vi "WPI_CameraSend Images To PC Loop_2Camera.vi"(8 "error in (no error)":errorcluster, 10 "CameraDevRef 2":T1, 11 "CameraDevRef":T1) -> ()   [LabVIEW 2015]
doc: "This VI is used to send images to the dashboard using the second enet port on the 8 slot controller. This is provided for compatibility, but is higher overhead than using the Camera MJPG approach.\n\nThis software is licensed. Open the labview\\readme\\WPI Robotics Library Open Source License.txt file for more information."
uses:
  <vilib>/Rock Robotics/WPI/Camera/WPI_CameraDevRef.ctl
  <vilib>/Rock Robotics/SystemInterfaces/NetworkCommunication/NetComm_UsageReport_ResourceType.ctl
  feed.vi
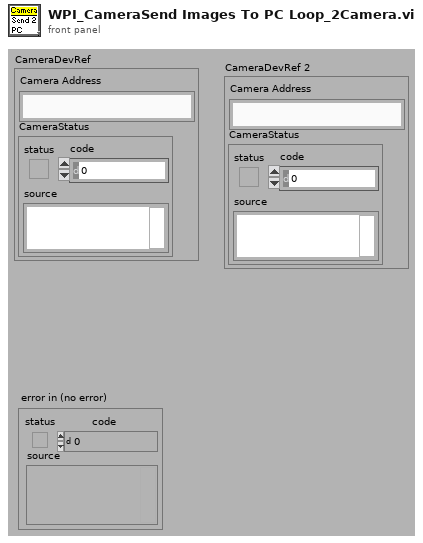
[diagram p1: front panel]
types:
  T1 = typedef "WPI_CameraDevRef.ctl" = cluster{"Camera Address":string, "CameraStatus":errorcluster}
  T2 = cluster{"fps":i32, "compression":i32, "compression 2":i32}
  T3 = typedef "NetComm_UsageReport_ResourceType.ctl" = enum8{"Controller", "Module", "Language", "CANPlugin", "Accelerometer", "ADXL345", "AnalogChannel", "AnalogTrigger", "AnalogTriggerOutput", "CANJaguar", "Compressor", "Counter", "Dashboard", "DigitalInput", "DigitalOutput", "DriverStationCIO", "DriverStationEIO", "DriverStationLCD", "Encoder", "GearTooth", "Gyro", "I2C", "Framework", "Jaguar", "Joystick", "Kinect", "KinectStick", "PIDController", "Preferences", "PWM", "Relay", "RobotDrive", "SerialPort", "Servo", "Solenoid", "SPI", "Task", "Ultrasonic", "Victor", "Button", "Command", "AxisCamera", "PCVideoServer", "SmartDashboard", "Talon", "HiTechnicColorSensor", "HiTechnicAccel", "HiTechnicCompass", "SRF08", "AnalogOutput", "Victor SP", "Talon SRX", "CAN Talon SRX", "ADXL362 Accel", "ADXRS450 Gyro", "Rev SPARK", "Mindsensors SD540", "Digital Filter"}
  T4 = enum16{"Update Mode", "Get Image", "Get Image Data"}
  T5 = typedef "Image Type" = u32
  T6 = typedef "IMAQ Image.ctl" = refnum<image>
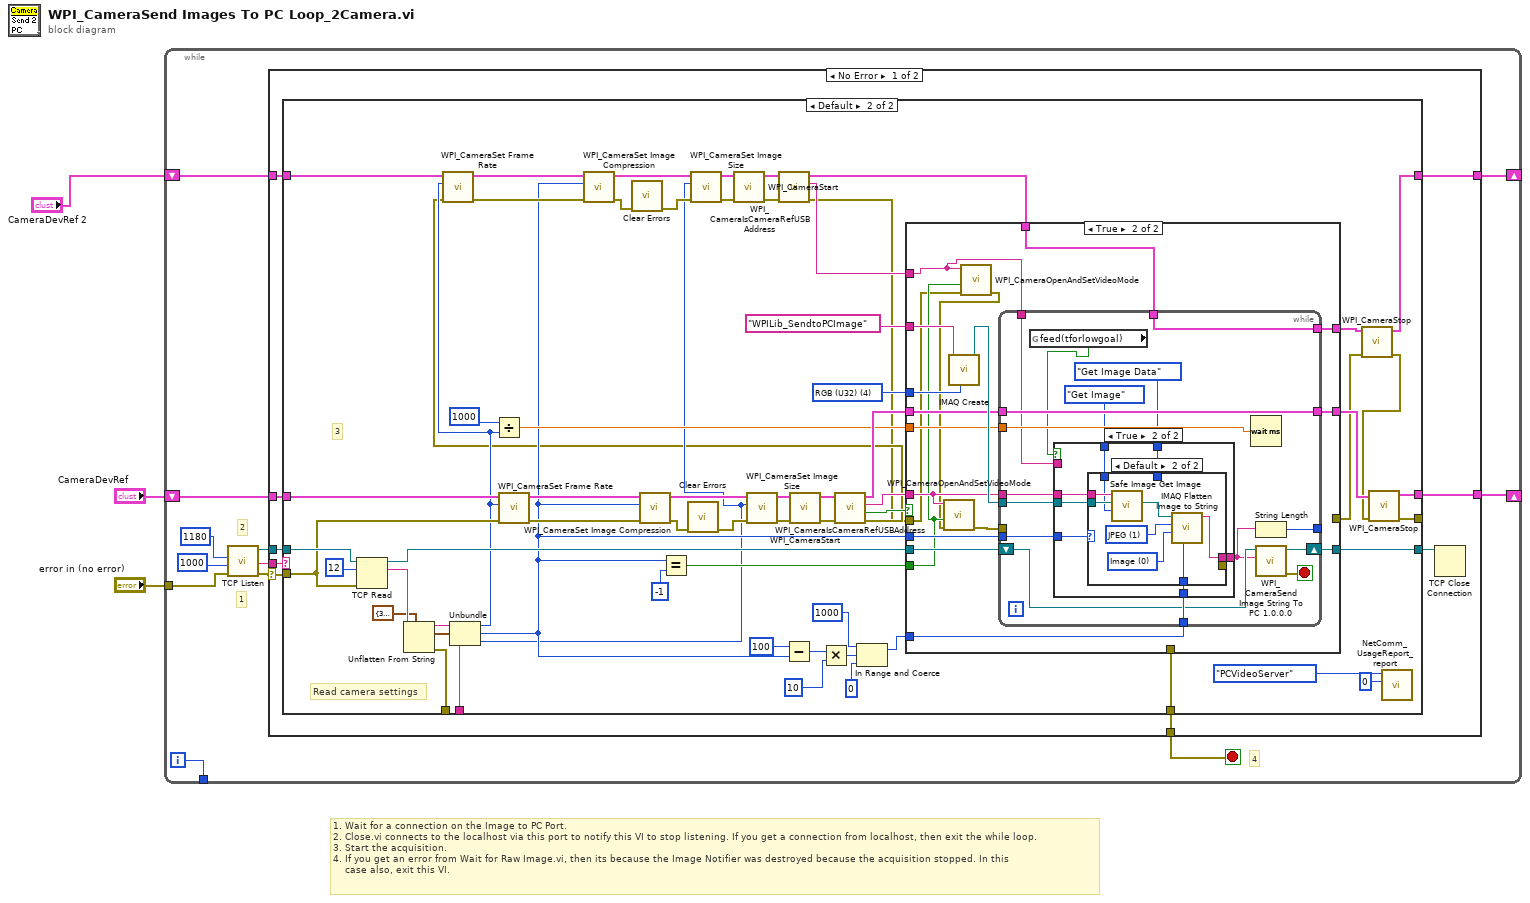
[diagram p0: block diagram]
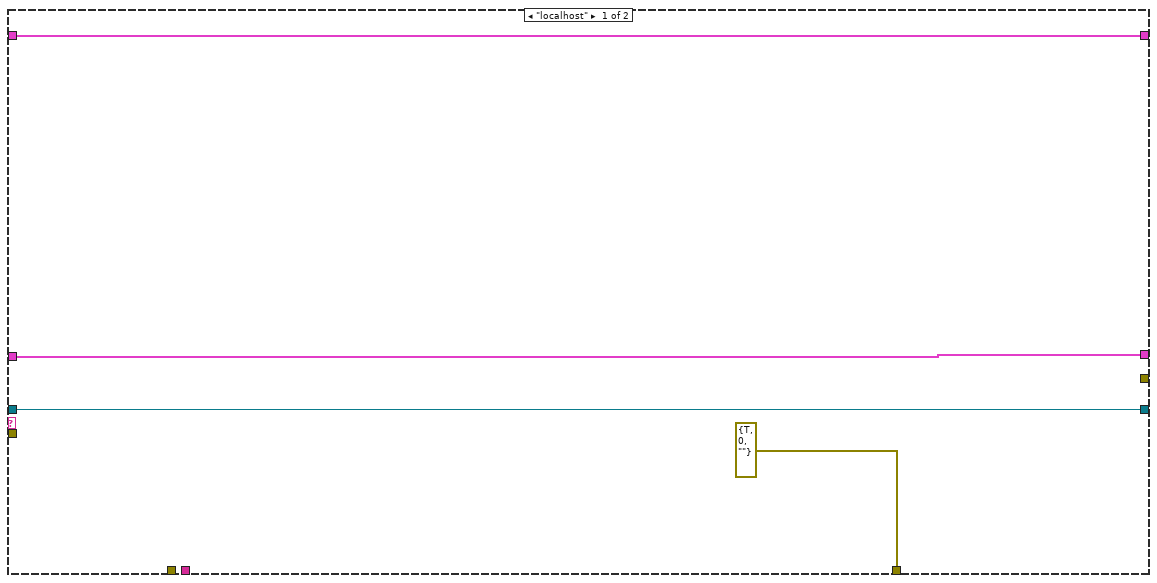
[diagram p2: hidden frame]
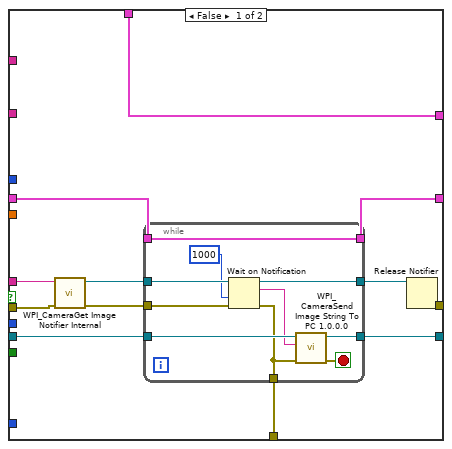
[diagram p3: hidden frame]
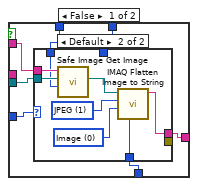
[diagram p4: hidden frame]
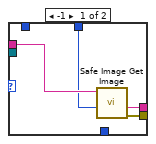
[diagram p5: hidden frame]
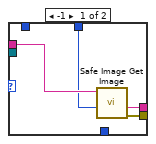
[diagram p6: hidden frame]
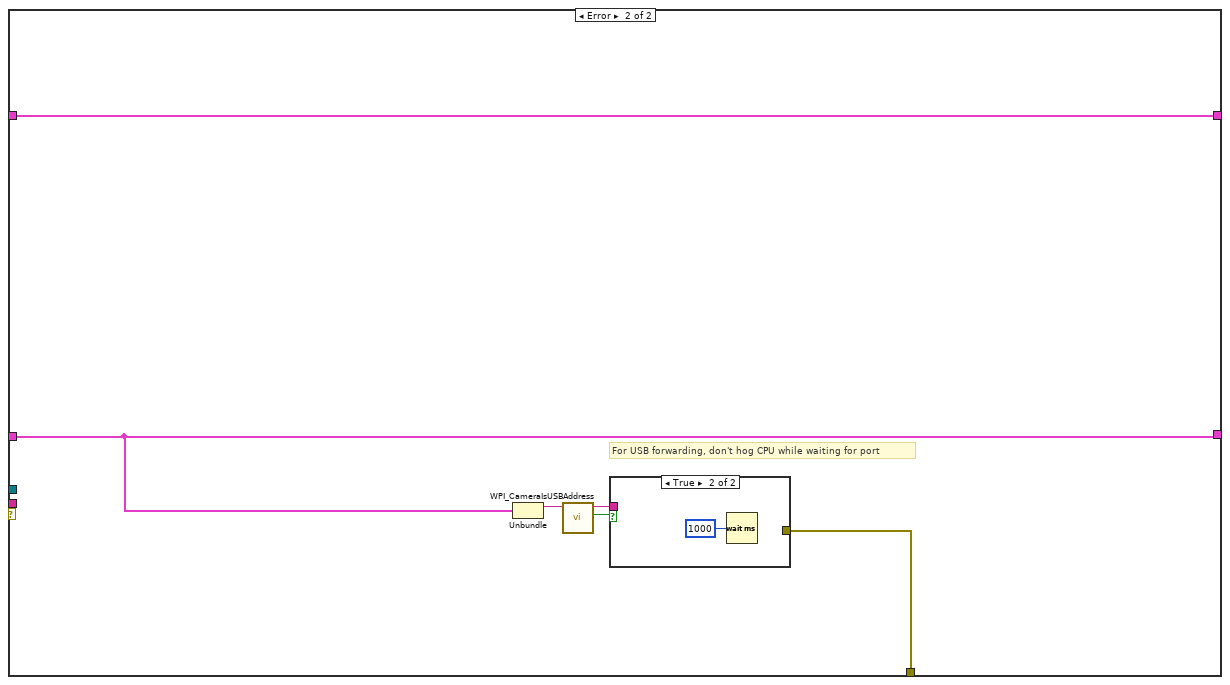
[diagram p7: hidden frame]
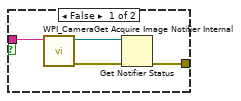
[diagram p8: hidden frame]
diagram:
  # "1. Wait for a connection on the Image to PC Port.\n2. Close.vi connects to the localhost via this port to notify this VI to stop listening. If you get a connection from localhost, then exit the while loop.\n3. Start the acquisition.\n4. If you get an error from Wait for Raw Image.vi, then its because the Image Notifier was destroyed because the acquisition stopped. In this\n    case also, exit this VI."
  n1 = while {
    tunnel: "error in (no error)" -> [w12]
    shift-right: [w15] -> _
    shift-left: "CameraDevRef" -> [w13]
    tunnel: [w6] -> _
    shift-right: [w4] -> _
    shift-left: "CameraDevRef 2" -> [w5]
    i -> [w6]
    stop <- w10 stop-if-true
    # "4"
    # "1"
    # "2"
    n2 = call <vilib>:"TCP Listen.vi"("error in (no error)"=w12, "timeout ms (wait forever: -1)"=u16 1000 ("port"), "port"=u16 1180) -> ("error out"=w8:errorcluster, "remote address"=w14:string, "connection ID"=w11:refnum<k5>)  [unwired: 1 in, 5 out]
    n3 = case shown="No Error" w8 {
      selector: w8 -> [w18 _]
      tunnel: [w24 w190] -> w15
      tunnel: w14 -> [w23 _]
      tunnel: w13 -> [w22 w190]
      tunnel: w11 -> [w21 _]
      tunnel: [w20 w191] -> w10
      tunnel: w5 -> [w17 w186]
      tunnel: [w16 w186] -> w4
      frame No Error {
        n4 = case shown="Default" w23 {
          tunnel: [w28 w89] -> w24
          tunnel: w22 -> [w28 w73]
          tunnel: w18 -> [_ w69]
          tunnel: w21 -> [w26 w77]
          tunnel: [errorcluster {"status"=TRUE, "code"=0, "source"=""} ("error out 2") w91] -> w20
          tunnel: [w26 w90] -> w19
          tunnel: [_ w88] -> _
          tunnel: [_ w51] -> _
          tunnel: [_ w50] -> _
          tunnel: w17 -> [w25 w40]
          tunnel: [w25 w33] -> w16
          frame "localhost" {
          }
          frame Default {
            w83 = T5 4 items=["Grayscale (U8)", "Grayscale (I16)", "Grayscale (SGL)", "Complex (CSG)", "RGB (U32)", "HSL (U32)", "RGB (U64)", "Grayscale (U16)"] ("Image Type")
            # "Read camera settings"
            # "3"
            n5 = TCP Read(connection ID=w77, bytes to read=12, error in (no error)=w69) -> (connection ID out=w76:refnum<k5>, data out=w74:string)  [unwired: 2 in, 1 out]
            n6 = Unflatten From String(type=T2 {"fps"=30, "compression"=32, "compression 2"=32} ("Camera Settings"), binary string=w74) -> (rest of the binary string=w50:string, value=w66:T2, error out=w51:errorcluster)  [unwired: 3 in]
            n7 = Unbundle(w66) -> ("fps"=w38:i32, "compression"=w39:i32, "compression 2"=w37:i32)
            n8 = Divide(x=u16 1000 ("port"), y=w38) -> (x/y=w64:dbl)
            n9 = call <vilib>:"WPI_CameraSet Frame Rate.vi"("error in (no error)"=w69, "Frame Rate (fps)"=w38, "CameraDevRef"=w73) -> ("error out"=w68:errorcluster, "CameraDevRef Out"=w72:T1)  [unwired: 7 in]
            n10 = call <vilib>:"WPI_CameraSet Image Compression.vi"("error in (no error)"=w68, "Compression"=w39, "CameraDevRef"=w72) -> ("error out"=w53:errorcluster, "CameraDevRef Out"=w71:T1)  [unwired: 7 in]
            n11 = Equal?(x=w39, y=-1) -> (x = y?=w54:bool)
            n12 = call <vilib>:"Clear Errors.vi"("error in (no error)"=w53) -> ("error out"=w52:errorcluster)  [unwired: 5 in, 1 out]
            n13 = call <vilib>:"WPI_CameraSet Image Size.vi"("error in (no error)"=w52, "Image Size"=w37, "CameraDevRef"=w71) -> ("error out"=w67:errorcluster, "CameraDevRef Out"=w70:T1)  [unwired: 7 in]
            n14 = Subtract(x=100, y=w39) -> (x-y=w59:i32)
            n15 = call <vilib>:"WPI_CameraStart.vi"("error in (no error)"=w67, "CameraDevRef"=w70) -> ("error out"=w80:errorcluster, "CameraDevRef"=w79:T1)  [unwired: 8 out]
            n16 = Multiply(x=w59, y=10) -> (x*y=w61:i32)
            n17 = call <vilib>:"WPI_CameraIsCameraRefUSBAddress.vi"("error in (no error)"=w80, "CameraDevRef"=w79) -> ("error out"=w32:errorcluster, "USB?"=w81:bool, "Camera Address Out"=w82:string, "CameraDevRef out"=w78:T1)  [unwired: 6 in]
            n18 = call <vilib>:"WPI_CameraSet Frame Rate.vi"("error in (no error)"=w32, "Frame Rate (fps)"=w38, "CameraDevRef"=w40) -> ("error out"=w46:errorcluster, "CameraDevRef Out"=w43:T1)  [unwired: 7 in]
            n19 = call <vilib>:"WPI_CameraSet Image Compression.vi"("error in (no error)"=w46, "Compression"=w39, "CameraDevRef"=w43) -> ("error out"=w48:errorcluster, "CameraDevRef Out"=w44:T1)  [unwired: 7 in]
            n20 = call <vilib>:"Clear Errors.vi"("error in (no error)"=w48) -> ("error out"=w49:errorcluster)  [unwired: 5 in, 1 out]
            n21 = call <vilib>:"WPI_CameraSet Image Size.vi"("error in (no error)"=w49, "Image Size"=w37, "CameraDevRef"=w44) -> ("error out"=w47:errorcluster, "CameraDevRef Out"=w45:T1)  [unwired: 7 in]
            n22 = call <vilib>:"WPI_CameraStart.vi"("error in (no error)"=w47, "CameraDevRef"=w45) -> ("error out"=w41:errorcluster, "CameraDevRef"=w42:T1)  [unwired: 8 out]
            n23 = call <vilib>:"WPI_CameraIsCameraRefUSBAddress.vi"("error in (no error)"=w41, "CameraDevRef"=w42) -> ("error out"=w31:errorcluster, "Camera Address Out"=w36:string, "CameraDevRef out"=w34:T1)  [unwired: 6 in, 1 out]
            n24 = In Range and Coerce(upper limit=1000, x=w61, lower limit=0) -> (coerced(x)=w57:i32)  [unwired: 1 out]
            n25 = case shown="True" w81 {
              tunnel: w76 -> [w103 w131]
              tunnel: [w102 _] -> w91
              tunnel: [w101 w130] -> w90
              tunnel: w31 -> [w100 w114]
              tunnel: w82 -> [w98 w121]
              tunnel: [w97 w125] -> w87
              tunnel: w78 -> [w96 w126]
              tunnel: [w94 _] -> w30
              tunnel: "WPILib_SendtoPCImage" -> [_ w128]
              tunnel: w83 -> [_ w127]
              tunnel: w57 -> [_ w124]
              tunnel: w64 -> [_ w123]
              tunnel: w39 -> [_ w122]
              tunnel: w54 -> [_ w116]
              tunnel: w36 -> [_ w119]
              tunnel: [w92 w118] -> w35
              tunnel: w34 -> [w92 w117]
              frame False {
                n26 = call <vilib>:"WPI_CameraGet Image Notifier Internal.vi"("error in (no error)"=w100, "Camera Address"=w98) -> ("error out"=w99:errorcluster, "Image Notifier"=w95:refnum<notifier>)  [unwired: 8 out]
                n27 = while {
                  tunnel: w99 -> [w109]
                  tunnel: w103 -> [w113]
                  tunnel: [w106] -> w102
                  tunnel: [w111] -> w101
                  tunnel: [w110] -> w97
                  tunnel: w96 -> [w110]
                  tunnel: w95 -> [w108]
                  tunnel: [w104] -> w93
                  stop <- w112 stop-if-true
                  n28 = Wait on Notification(notifier=w108, timeout in ms (-1)=1000 ("Timeout in ms (-1)"), error in (no error)=w109) -> (notifier out=w104:refnum<notifier>, notification=w107:string, error out=w106:errorcluster)  [unwired: 2 out]
                  n29 = call <vilib>:"WPI_CameraSend Image String To PC 1.0.0.0.vi"("error in (no error)"=w106, "String"=w107, "TCP Connection ID"=w113) -> ("error out"=w112:errorcluster, "TCP Connection ID out"=w111:refnum<k5>)  [unwired: 7 out]
                }
                n30 = Release Notifier(notifier=w93) -> (error out=w94:errorcluster)  [unwired: 1 in, 3 out]
              }
              frame True {
                n31 = call "IMAQ Create"("Image Name"=w128, "Image Type"=w127) -> ("New Image"=w129:T6)  [unwired: 3 in, 1 out]
                n32 = call <vilib>:"WPI_CameraOpenAndSetVideoMode.vi"("error in (no error)"=w114, "USB JPEG"=w116, "Camera Address Out"=w119) -> ("error out"=w115:errorcluster)  [unwired: 8 in]
                n33 = call <vilib>:"WPI_CameraOpenAndSetVideoMode.vi"("error in (no error)"=w115, "USB JPEG"=w116, "Camera Address Out"=w121) -> ("error out"=w120:errorcluster)  [unwired: 8 in]
                n34 = while {
                  tunnel: w121 -> [w146]
                  shift-right: [w147] -> w130
                  shift-left: w131 -> [w140]
                  tunnel: w129 -> [w145]
                  tunnel: [w143] -> w125
                  tunnel: w126 -> [w143]
                  tunnel: w124 -> [w142]
                  tunnel: w123 -> [w141]
                  tunnel: [w138] -> _
                  tunnel: w122 -> [w137]
                  tunnel: w120 -> [_]
                  tunnel: w119 -> [w134]
                  tunnel: [w133] -> w118
                  tunnel: w117 -> [w133]
                  stop <- w144 stop-if-true
                  n35 = global read "feed.vi" "feed(tforlowgoal)"() -> (w132:bool)
                  n36 = case shown="True" w132 {
                    tunnel: w146 -> [_ w173]
                    tunnel: w145 -> [w151 w172]
                    tunnel: w142 -> [w153 w171]
                    tunnel: [w154 w170] -> w139
                    tunnel: w137 -> [w152 w169]
                    tunnel: T4."Get Image Data" ("Operation") -> [w148 w168]
                    tunnel: T4."Get Image" ("Operation") -> [w149 w167]
                    tunnel: w134 -> [w150 _]
                    frame False {
                      n37 = case shown="Default" w152 {
                        tunnel: [w157 w166] -> w154
                        tunnel: w150 -> [w158 w162]
                        tunnel: w151 -> [_ w161]
                        tunnel: w153 -> [_ w163]
                        tunnel: [w156 _] -> _
                        tunnel: w148 -> [w155 _]
                        tunnel: w149 -> [_ w159]
                        frame -1 {
                          n38 = call <vilib>:"Safe Image Get Image.vi"("Operation"=w155, "Session In"=w158) -> ("error out"=w156:errorcluster, "Image Data String"=w157:string)  [unwired: 6 in, 2 out]
                        }
                        frame Default {
                          w164 = 0 items=["Image", "Image and Vision Info", "Reference to Image"] ("Type of Flatten (Image and Vision Info)")
                          w165 = 1 items=["None", "JPEG", "PACKED BINARY"] ("Compression (None)")
                          n39 = call <vilib>:"Safe Image Get Image.vi"("Operation"=w159, "Image In"=w161, "Session In"=w162) -> ("Image Out"=w160:T6)  [unwired: 5 in, 3 out]
                          n40 = call "IMAQ Flatten Image to String"("Quality (750)"=w163, "Type of Flatten (Image and Vision Info)"=w164, "Compression (None)"=w165, "Image"=w160) -> ("Data String"=w166:string)  [unwired: 6 in, 1 out]
                        }
                      }
                    }
                    frame True {
                      n41 = case shown="Default" w169 {
                        tunnel: [w176 w185] -> w170
                        tunnel: w173 -> [w177 w181]
                        tunnel: w172 -> [_ w180]
                        tunnel: w171 -> [_ w182]
                        tunnel: [w175 _] -> _
                        tunnel: w168 -> [w174 _]
                        tunnel: w167 -> [_ w178]
                        frame -1 {
                          n42 = call <vilib>:"Safe Image Get Image.vi"("Operation"=w174, "Session In"=w177) -> ("error out"=w175:errorcluster, "Image Data String"=w176:string)  [unwired: 6 in, 2 out]
                        }
                        frame Default {
                          w183 = 0 items=["Image", "Image and Vision Info", "Reference to Image"] ("Type of Flatten (Image and Vision Info)")
                          w184 = 1 items=["None", "JPEG", "PACKED BINARY"] ("Compression (None)")
                          n43 = call <vilib>:"Safe Image Get Image.vi"("Operation"=w178, "Image In"=w180, "Session In"=w181) -> ("Image Out"=w179:T6)  [unwired: 5 in, 3 out]
                          n44 = call "IMAQ Flatten Image to String"("Quality (750)"=w182, "Type of Flatten (Image and Vision Info)"=w183, "Compression (None)"=w184, "Image"=w179) -> ("Data String"=w185:string)  [unwired: 6 in, 1 out]
                        }
                      }
                    }
                  }
                  n45 = Wait (ms)(milliseconds to wait=w141) -> ()  [unwired: 1 out]
                  n46 = String Length(string=w139) -> (length=w138:i32)
                  n47 = call <vilib>:"WPI_CameraSend Image String To PC 1.0.0.0.vi"("String"=w139, "TCP Connection ID"=w140) -> ("error out"=w144:errorcluster, "TCP Connection ID out"=w147:refnum<k5>)  [unwired: 1 in, 7 out]
                }
              }
            }
            n48 = call <vilib>:"WPI_CameraStop.vi"("error in (no error)"=w30, "CameraDevRef"=w35) -> ("error out"=w29:errorcluster, "CameraDevRef"=w33:T1)  [unwired: 8 out]
            n49 = call <vilib>:"WPI_CameraStop.vi"("error in (no error)"=w29, "CameraDevRef"=w87) -> ("error out"=w88:errorcluster, "CameraDevRef"=w89:T1)  [unwired: 8 out]
            n50 = call <vilib>:"NetComm_UsageReport_report.vi"("Instance Number"=u8 0, "Resource Type"=NetComm_UsageReport_ResourceType."PCVideoServer") -> ()  [unwired: 10 in]
          }
        }
        n51 = TCP Close Connection(connection ID=w19) -> ()  [unwired: 1 in, 3 out]
      }
      frame Error {
        # "For USB forwarding, don't hog CPU while waiting for port"
        n52 = Unbundle(w190) -> ("Camera Address"=w189:string)  [unwired: 1 out]
        n53 = call <vilib>:"WPI_CameraIsUSBAddress.vi"("Camera Address In"=w189) -> ("USB?"=w187:bool, "Camera Address Out"=w188:string)  [unwired: 8 in, 1 out]
        n54 = case shown="True" w187 {
          tunnel: [w195 _] -> w191
          tunnel: w188 -> [w192 _]
          frame False {
            n55 = call <vilib>:"WPI_CameraGet Acquire Image Notifier Internal.vi"("Camera Address"=w192) -> ("error out"=w193:errorcluster, "Acquire Image Notifier"=w194:refnum<notifier>)  [unwired: 1 in, 8 out]
            n56 = Get Notifier Status(notifier=w194, error in (no error)=w193) -> (error out=w195:errorcluster)  [unwired: 4 out]
          }
          frame True {
            n57 = Wait (ms)(milliseconds to wait=u32 1000) -> ()  [unwired: 1 out]
          }
        }
      }
    }
  }
